vi "DN4_ControlEndTask.vi"(2 "error in (no error)":errorcluster, 3 "Task ID":u32) -> (0 "error out":errorcluster, 1 "Task ID":u32)   [LabVIEW 2009]
doc: "finish the task to do clean up work"
uses:
  Windows/System32/AdvLvDaq.dll
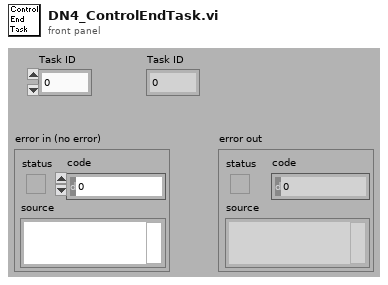
[diagram p1: front panel]
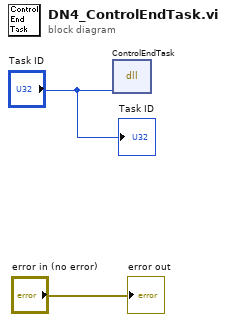
[diagram p0: block diagram]
diagram:
  n1 = dll-call lib="C:/Windows/System32/AdvLvDaq.dll" fn="ControlEndTask"("taskId"="Task ID") -> ()  [unwired: 4 in, 3 out]
  "Task ID" <- "Task ID"
  "error out" <- "error in (no error)"
